vi "one_button.vi"(7 "callee":refnum<vi>, 8 "error in (no error)":errorcluster, 10 "configuration":T1, 11 "v1 in":refnum<class "v1.lvclass">) -> (0 "error out":errorcluster, 2 "dialog_selection":T2, 3 "v1 out":refnum<class "v1.lvclass">)   [LabVIEW 2015, in "lv-dialog.lvlib" / "v1.lvlib" / "v1.lvclass"]
uses:
  v1.lvclass
  _controls/selection.ctl
  v1.lvlib
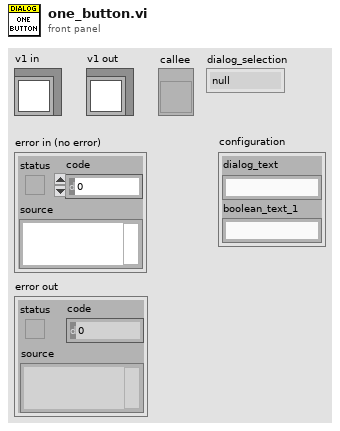
[diagram p1: front panel]
types:
  T1 = cluster{"dialog_text":string, "boolean_text_1":string}
  T2 = typedef "lv-dialog.lvlib/v1.lvlib/selection.ctl" = enum16{"null", "panel_closed", "button_1", "button_2", "button_3", "cancelled"}
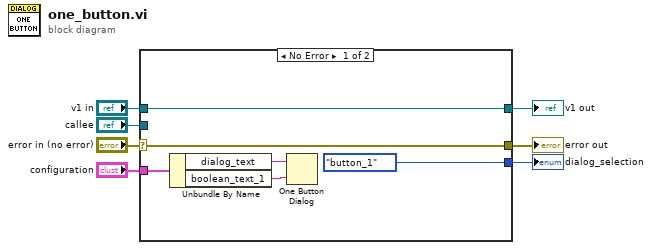
[diagram p0: block diagram]
diagram:
  n1 = case shown="No Error" "error in (no error)" {
    selector: "error in (no error)" -> [w9 w15]
    tunnel: [w9 w15] -> w6
    tunnel: [w13 w14] -> w4
    tunnel: "v1 in" -> [w13 w14]
    tunnel: "callee" -> [_ _]
    tunnel: "configuration" -> [w12 _]
    tunnel: [selection."button_1" ("dialog_selection") _] -> w1
    frame No Error {
      n2 = Unbundle By Name(w12) -> ("dialog_text"=w11:string, "boolean_text_1"=w10:string)
      n3 = One Button Dialog(message=w11, button name ("OK")=w10) -> ()  [unwired: 1 out]
    }
    frame Error {
    }
  }
  "error out" <- w6
  "v1 out" <- w4
  "dialog_selection" <- w1
